vi "Query.vi"(8 "error in (no error)":errorcluster, 9 "Parameters":map{string, variant}(c390), 10 "Query":string, 11 "Sqlite Database Manager in":refnum<class "Sqlite Database Manager.lvclass">) -> (0 "error out":errorcluster, 1 "Rows":map{string, variant}[](array[numeric]), 3 "Sqlite Database Manager out":refnum<class "Sqlite Database Manager.lvclass">)   [LabVIEW 2019, in "HierDAL Library.lvlib" / "Database.lvlib" / "Sqlite Database Manager.lvclass"]
doc: "Executes a SQL query and retrieves the results.\nParameters are used to safely inject values into the SQL command, preventing SQL injection attacks.\nIt ensure that inputs are only ever treated as literal values and never executed.\n\nParameters can be prefixed with either :, @, or $.\ne.g.\n\"\"\"\n SELECT country, year \n FROM generals\n WHERE name = @name\n\"\"\"\n\n<b>Query</b> - The SQL query to execute.\n<b>Parameters</b> - A map of parameter (must have prefix) names and their corresponding values.\n<b>Rows</b> - A list of maps, each representing a row with column-value pairs."
uses:
  Sqlite Database Manager.lvclass
  Sqlite Database Manager.lvclass/Sqlite Database Manager.ctl
  System.Data.SQLite
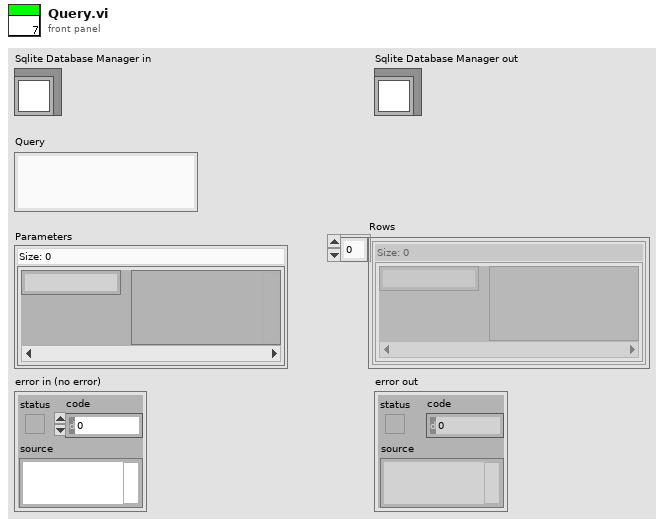
[diagram p1: front panel]
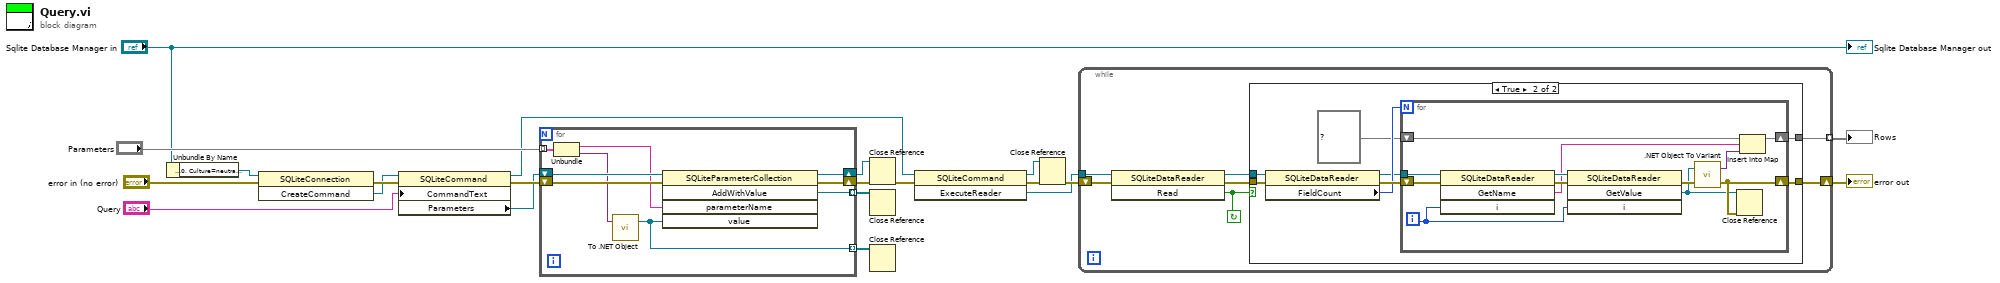
[diagram p0: block diagram]
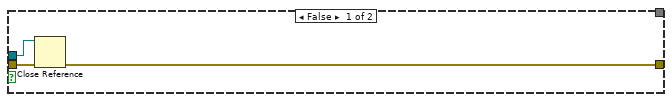
[diagram p2: hidden frame]
diagram:
  n1 = Unbundle By Name("Sqlite Database Manager in") -> ("Connection"=w21:refnum<k24>)
  n2 = invoke class="SQLiteConnection" method="CreateCommand"(reference=w21, error in="error in (no error)") -> (error out=w19:errorcluster, "CreateCommand"=w18:refnum<k24>)  [unwired: 1 in, 1 out]
  n3 = property class="SQLiteCommand"(reference=w18, error in=w19, "CommandText"="Query") -> (reference out=w8:refnum<k24>, error out=w16:errorcluster, "Parameters"=w15:refnum<k24>)
  n4 = for {
    shift-right: [w26] -> w10
    shift-left: w15 -> [w28]
    tunnel: "Parameters" -> [w29] mode=indexing
    shift-right: [w27] -> w13
    shift-left: w16 -> [w30]
    tunnel: [w25] -> w11 mode=indexing
    tunnel: [w24] -> w12 mode=indexing
    n5 = Unbundle(w29) -> ("Parameter"=w22:string, "Value"=w23:variant)
    n6 = call <vilib>:"To .NET Object.vi"("anything"=w23) -> (".NET object"=w24:refnum<k24>)  [unwired: 1 in, 1 out]
    n7 = invoke class="SQLiteParameterCollection" method="AddWithValue"(reference=w28, error in=w30, "parameterName"=w22, "value"=w24) -> (reference out=w26:refnum<k24>, error out=w27:errorcluster, "AddWithValue"=w25:refnum<k24>)  [unwired: 1 in, 2 out]
  }
  n8 = Close Reference(reference=w10, error in (no error)=w13) -> (error out=w9:errorcluster)
  n9 = Close Reference(reference=w11) -> ()  [unwired: 1 in, 1 out]
  n10 = Close Reference(reference=w12) -> ()  [unwired: 1 in, 1 out]
  n11 = invoke class="SQLiteCommand" method="ExecuteReader"(reference=w8, error in=w9) -> (reference out=w6:refnum<k24>, error out=w7:errorcluster, "ExecuteReader"=w4:refnum<k24>)  [unwired: 1 in]
  n12 = Close Reference(reference=w6, error in (no error)=w7) -> (error out=w5:errorcluster)
  n13 = while {
    shift-right: [w32] -> w3
    shift-left: w5 -> [w37]
    tunnel: w4 -> [w36]
    tunnel: [w31] -> w2 mode=indexing
    stop <- w35 continue-if-true
    n14 = invoke class="SQLiteDataReader" method="Read"(reference=w36, error in=w37) -> (reference out=w33:refnum<k24>, error out=w34:errorcluster, "Read"=w35:bool)  [unwired: 1 in]
    n15 = case shown="True" w35 {
      tunnel: w34 -> [w40 w48]
      tunnel: w33 -> [w39 w47]
      tunnel: [w38 w42] -> w32
      tunnel: [_ w43] -> w31
      frame False {
        n16 = Close Reference(reference=w39, error in (no error)=w40) -> (error out=w38:errorcluster)
      }
      frame True {
        n17 = property class="SQLiteDataReader"(reference=w47, error in=w48) -> (reference out=w41:refnum<k24>, error out=w46:errorcluster, "FieldCount"=w45:i32)
        n18 = for {
          N: w45 -> [_]
          shift-right: [w55] -> w42
          shift-left: w46 -> [w60]
          shift-right: [w52] -> w43
          shift-left: map{string, variant} {} ("Row") -> [w53]
          tunnel: w41 -> [w59]
          i -> [w57]
          n19 = invoke class="SQLiteDataReader" method="GetName"(reference=w59, error in=w60, "i"=w57) -> (reference out=w51:refnum<k24>, error out=w58:errorcluster, "GetName"=w50:string)  [unwired: 1 in, 1 out]
          n20 = invoke class="SQLiteDataReader" method="GetValue"(reference=w51, error in=w58, "i"=w57) -> (error out=w56:errorcluster, "GetValue"=w54:refnum<k24>)  [unwired: 1 in, 2 out]
          n21 = call <vilib>:".NET Object To Variant.vi"("error in (no error)"=w56, ".NET object"=w54) -> ("error out"=w55:errorcluster, "variant"=w49:variant)
          n22 = Close Reference(reference=w54, error in (no error)=w55) -> ()  [unwired: 1 out]
          n23 = Insert Into Map(map in=w53, key=w50, value=w49) -> (map out=w52:map{string, variant})  [unwired: 2 out]
        }
      }
    }
  }
  "error out" <- w3
  "Rows" <- w2
  "Sqlite Database Manager out" <- "Sqlite Database Manager in"
